vi "Remove Sheet.vi"(8 "error in (no error)":errorcluster, 10 "Sheet Name":string, 11 "MS-Excel in":refnum<class "MS-Excel.lvclass">) -> (0 "error out":errorcluster, 3 "MS-Excel out":refnum<class "MS-Excel.lvclass">)   [LabVIEW 2017, in "LabVIEW NPOI.lvlib" / "MS-Excel.lvclass"]
doc: "Removes sheet with the given <b>Sheet Name</b> from the associated workbook to the <b>Document</b>.\n\nThis method makes sure that if the removed sheet was active, another sheet will become active in its place. Furthermore, if the removed sheet was the only selected sheet, another sheet will become selected. The newly active/selected sheet will have the same index, or one less if the removed sheet was the last in the workbook."
uses:
  MS-Excel.lvclass
  Get Current SheetIndex.vi
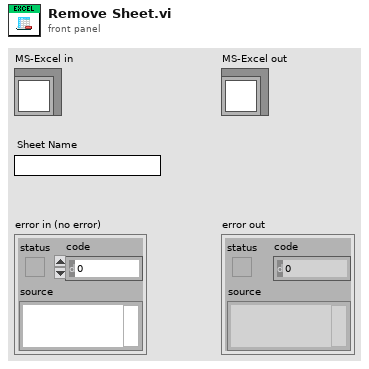
[diagram p1: front panel]
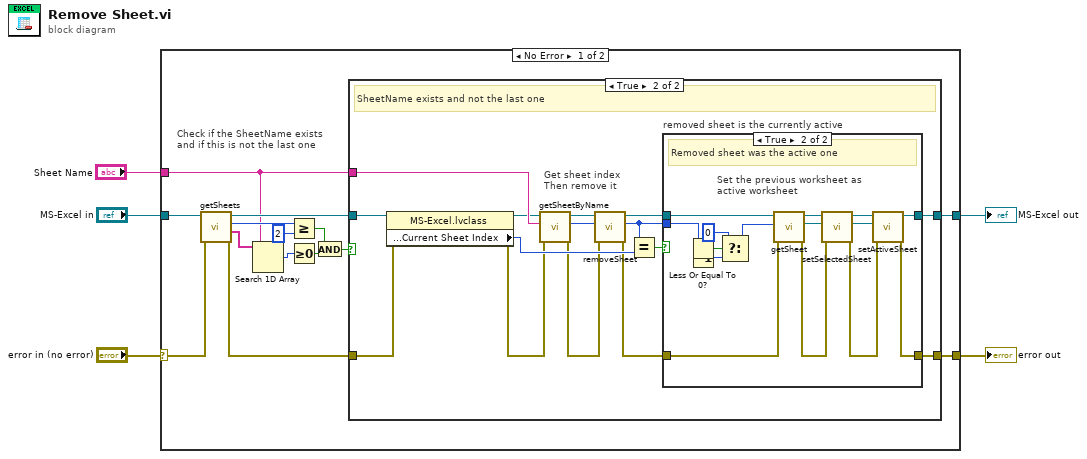
[diagram p0: block diagram]
diagram:
  n1 = case shown="No Error" "error in (no error)" {
    selector: "error in (no error)" -> [w18 w53]
    tunnel: [w10 w53] -> w4
    tunnel: [w16 w52] -> w2
    tunnel: "MS-Excel in" -> [w19 w52]
    tunnel: "Sheet Name" -> [w8 _]
    frame No Error {
      # "Check if the SheetName exists and if this is not the last one"
      n2 = call-dynamic "getSheets.vi"("error in (no error)"=w18, "MS-Excel in"=w19) -> ("error out"=w9:errorcluster, "Sheet Names"=w6:string[], "#Sheets"=w15:i32, "MS-Excel out"=w17:refnum<class "MS-Excel.lvclass">)  [unwired: 6 in]
      n3 = Search 1D Array(1D array=w6, element=w8) -> (index of element=w7:i32)  [unwired: 1 in]
      n4 = Greater Or Equal?(x=w15, y=2) -> (x >= y?=w13:bool)
      n5 = Greater Or Equal To 0?(x=w7) -> (x >= 0?=w12:bool)
      n6 = And(x=w13, y=w12) -> (x .and. y?=w11:bool)
      n7 = case shown="True" w11 {
        tunnel: w17 -> [w21 w29]
        tunnel: [w21 w35] -> w16
        tunnel: [w20 w34] -> w10
        tunnel: w9 -> [w20 w25]
        tunnel: w8 -> [_ w33]
        frame False {
          # "SheetName is not in the Sheet List or is the last sheet"
        }
        frame True {
          # "Get sheet index\nThen remove it"
          # "SheetName exists and not the last one"
          n8 = property class="MS-Excel.lvclass"(reference=w29, error in=w25) -> (reference out=w28:refnum<class "MS-Excel.lvclass">, error out=w24:errorcluster, "Public VIs:Properties:Current Sheet Index"=w32:i32)
          n9 = call-dynamic "getSheetByName.vi"("error in (no error)"=w24, "Sheet Name"=w33, "MS-Excel in"=w28) -> ("error out"=w23:errorcluster, "SheetIndex"=w31:i32, "MS-Excel out"=w27:refnum<class "MS-Excel.lvclass">)  [unwired: 5 in, 1 out]
          n10 = call-dynamic "removeSheet.vi"("error in (no error)"=w23, "Sheet Index"=w31, "MS-Excel in"=w27) -> ("error out"=w22:errorcluster, "MS-Excel out"=w26:refnum<class "MS-Excel.lvclass">)  [unwired: 7 in]
          n11 = Equal?(x=w31, y=w32) -> (x = y?=w30:bool)
          n12 = case "removed sheet is the currently active" shown="True" w30 {
            tunnel: w22 -> [w36 w51]
            tunnel: [w37 w50] -> w35
            tunnel: [w36 w49] -> w34
            tunnel: w26 -> [w37 w48]
            tunnel: w31 -> [_ w40]
            frame False {
              # "Another sheet is the active one"
            }
            frame True {
              # "Set the previous worksheet as active worksheet"
              # "Removed sheet was the active one"
              n13 = Less Or Equal To 0?(x=w40) -> (x <= 0?=w42:bool)
              n14 = Decrement(x=w40) -> (x-1=w39:i32)
              n15 = Select(t=0, s=w42, f=w39) -> (s? t:f=w38:i32)
              n16 = call-dynamic "getSheet.vi"("error in (no error)"=w51, "Sheet Index"=w38, "MS-Excel in"=w48) -> ("error out"=w45:errorcluster, "Sheet Ref"=w44:refnum<k24>, "MS-Excel out"=w47:refnum<class "MS-Excel.lvclass">)  [unwired: 6 in]
              n17 = call-dynamic "setSelectedSheet.vi"("error in (no error)"=w45, "Sheet Ref"=w44, "MS-Excel in"=w47) -> ("error out"=w43:errorcluster, "MS-Excel out"=w46:refnum<class "MS-Excel.lvclass">)  [unwired: 7 in]
              n18 = call-dynamic "setActiveSheet.vi"("error in (no error)"=w43, "Sheet Ref"=w44, "MS-Excel in"=w46) -> ("error out"=w49:errorcluster, "MS-Excel out"=w50:refnum<class "MS-Excel.lvclass">)  [unwired: 7 in]
            }
          }
        }
      }
    }
    frame Error {
    }
  }
  "error out" <- w4
  "MS-Excel out" <- w2
